vi "CSTK_Button_Icon_Dialog_Configuration.vi"(11 "State in":T1={"ButtonSize"={"False"={"Width"=0, "Height"=0}, "True"={"Width"=0, "Height"=0}, "True to False"={"Width"=0, "Height"=0}, "False to True"={"Width"=0, "Height"=0}, "Hover in False"={"Width"=0, "Height"=0}, "Hover in True"={"Width"=0, "Height"=0}}, "Logo Image"={"False"={"image type"=0, "image depth"=0, "image"=[], "mask"=[], "colors"=[], "Rectangle"={"left"=0, "top"=0, "right"=0, "bottom"=0}}, "True"={"image type"=0, "image depth"=0, "image"=[], "mask"=[], "colors"=[], "Rectangle"={"left"=0, "top"=0, "right"=0, "bottom"=0}}, "True to False"={"image type"=0, "image depth"=0, "image"=[], "mask"=[], "colors"=[], "Rectangle"={"left"=0, "top"=0, "right"=0, "bottom"=0}}, "False to True"={"image type"=0, "image depth"=0, "image"=[], "mask"=[], "colors"=[], "Rectangle"={"left"=0, "top"=0, "right"=0, "bottom"=0}}, "Hover in False"={"image type"=0, "image depth"=0, "image"=[], "mask"=[], "colors"=[], "Rectangle"={"left"=0, "top"=0, "right"=0, "bottom"=0}}, "Hover in True"={"image type"=0, "image depth"=0, "image"=[], "mask"=[], "colors"=[], "Rectangle"={"left"=0, "top"=0, "right"=0, "bottom"=0}}}, "Logo Properties"={"False"={"Display Logo?"=FALSE, "Horizontal Offset"=0}, "True"={"Display Logo?"=FALSE, "Horizontal Offset"=0}, "True to False"={"Display Logo?"=FALSE, "Horizontal Offset"=0}, "False to True"={"Display Logo?"=FALSE, "Horizontal Offset"=0}, "Hover in False"={"Display Logo?"=FALSE, "Horizontal Offset"=0}, "Hover in True"={"Display Logo?"=FALSE, "Horizontal Offset"=0}}, "Text String"={"False"="", "True"="", "True to False"="", "False to True"="", "Hover in False"="", "Hover in True"=""}, "Text Properties"={"False"={"Display Text?"=FALSE, "Text Color"=0, "Horizontal Offset"=0, "Font Style"={"Font Name"="", "Size"=0, "Strikeout?"=FALSE, "Italic?"=FALSE, "Underline?"=FALSE, "Outline?"=FALSE, "Shadow?"=FALSE, "Bold?"=FALSE}}, "True"={"Display Text?"=FALSE, "Text Color"=0, "Horizontal Offset"=0, "Font Style"={"Font Name"="", "Size"=0, "Strikeout?"=FALSE, "Italic?"=FALSE, "Underline?"=FALSE, "Outline?"=FALSE, "Shadow?"=FALSE, "Bold?"=FALSE}}, "True to False"={"Display Text?"=FALSE, "Text Color"=0, "Horizontal Offset"=0, "Font Style"={"Font Name"="", "Size"=0, "Strikeout?"=FALSE, "Italic?"=FALSE, "Underline?"=FALSE, "Outline?"=FALSE, "Shadow?"=FALSE, "Bold?"=FALSE}}, "False to True"={"Display Text?"=FALSE, "Text Color"=0, "Horizontal Offset"=0, "Font Style"={"Font Name"="", "Size"=0, "Strikeout?"=FALSE, "Italic?"=FALSE, "Underline?"=FALSE, "Outline?"=FALSE, "Shadow?"=FALSE, "Bold?"=FALSE}}, "Hover in False"={"Display Text?"=FALSE, "Text Color"=0, "Horizontal Offset"=0, "Font Style"={"Font Name"="", "Size"=0, "Strikeout?"=FALSE, "Italic?"=FALSE, "Underline?"=FALSE, "Outline?"=FALSE, "Shadow?"=FALSE, "Bold?"=FALSE}}, "Hover in True"={"Display Text?"=FALSE, "Text Color"=0, "Horizontal Offset"=0, "Font Style"={"Font Name"="", "Size"=0, "Strikeout?"=FALSE, "Italic?"=FALSE, "Underline?"=FALSE, "Outline?"=FALSE, "Shadow?"=FALSE, "Bold?"=FALSE}}}, "BG Color"={"False"=0, "True"=0, "True to False"=0, "False to True"=0, "Hover in False"=0, "Hover in True"=0}, "Border Color"={"False"=0, "True"=0, "True to False"=0, "False to True"=0, "Hover in False"=0, "Hover in True"=0}, "Border Properties"={"False"={"Radius"=0, "Border Style"={"Width"=3, "Style"=enum."Solid"}}, "True"={"Radius"=0, "Border Style"={"Width"=3, "Style"=enum."Solid"}}, "True to False"={"Radius"=0, "Border Style"={"Width"=3, "Style"=enum."Solid"}}, "False to True"={"Radius"=0, "Border Style"={"Width"=3, "Style"=enum."Solid"}}, "Hover in False"={"Radius"=0, "Border Style"={"Width"=3, "Style"=enum."Solid"}}, "Hover in True"={"Radius"=0, "Border Style"={"Width"=3, "Style"=enum."Solid"}}}, "Current BG Image"={"False"=bytes[0], "True"=bytes[0], "True to False"=bytes[0], "False to True"=bytes[0], "Hover in False"=bytes[0], "Hover in True"=bytes[0]}, "DrawAreaSize"={"False"={"Width"=0, "Height"=0}, "True"={"Width"=0, "Height"=0}, "True to False"={"Width"=0, "Height"=0}, "False to True"={"Width"=0, "Height"=0}, "Hover in False"={"Width"=0, "Height"=0}, "Hover in True"={"Width"=0, "Height"=0}}, "Text String Offset"={"False"=0, "True"=0, "True to False"=0, "False to True"=0, "Hover in False"=0, "Hover in True"=0}} caption="状态") -> (1 "Action Name":string, 2 "State Changed?":bool, 3 "State out":T1={"ButtonSize"={"False"={"Width"=0, "Height"=0}, "True"={"Width"=0, "Height"=0}, "True to False"={"Width"=0, "Height"=0}, "False to True"={"Width"=0, "Height"=0}, "Hover in False"={"Width"=0, "Height"=0}, "Hover in True"={"Width"=0, "Height"=0}}, "Logo Image"={"False"={"image type"=0, "image depth"=0, "image"=[], "mask"=[], "colors"=[], "Rectangle"={"left"=0, "top"=0, "right"=0, "bottom"=0}}, "True"={"image type"=0, "image depth"=0, "image"=[], "mask"=[], "colors"=[], "Rectangle"={"left"=0, "top"=0, "right"=0, "bottom"=0}}, "True to False"={"image type"=0, "image depth"=0, "image"=[], "mask"=[], "colors"=[], "Rectangle"={"left"=0, "top"=0, "right"=0, "bottom"=0}}, "False to True"={"image type"=0, "image depth"=0, "image"=[], "mask"=[], "colors"=[], "Rectangle"={"left"=0, "top"=0, "right"=0, "bottom"=0}}, "Hover in False"={"image type"=0, "image depth"=0, "image"=[], "mask"=[], "colors"=[], "Rectangle"={"left"=0, "top"=0, "right"=0, "bottom"=0}}, "Hover in True"={"image type"=0, "image depth"=0, "image"=[], "mask"=[], "colors"=[], "Rectangle"={"left"=0, "top"=0, "right"=0, "bottom"=0}}}, "Logo Properties"={"False"={"Display Logo?"=FALSE, "Horizontal Offset"=0}, "True"={"Display Logo?"=FALSE, "Horizontal Offset"=0}, "True to False"={"Display Logo?"=FALSE, "Horizontal Offset"=0}, "False to True"={"Display Logo?"=FALSE, "Horizontal Offset"=0}, "Hover in False"={"Display Logo?"=FALSE, "Horizontal Offset"=0}, "Hover in True"={"Display Logo?"=FALSE, "Horizontal Offset"=0}}, "Text String"={"False"="", "True"="", "True to False"="", "False to True"="", "Hover in False"="", "Hover in True"=""}, "Text Properties"={"False"={"Display Text?"=FALSE, "Text Color"=0, "Horizontal Offset"=0, "Font Style"={"Font Name"="", "Size"=0, "Strikeout?"=FALSE, "Italic?"=FALSE, "Underline?"=FALSE, "Outline?"=FALSE, "Shadow?"=FALSE, "Bold?"=FALSE}}, "True"={"Display Text?"=FALSE, "Text Color"=0, "Horizontal Offset"=0, "Font Style"={"Font Name"="", "Size"=0, "Strikeout?"=FALSE, "Italic?"=FALSE, "Underline?"=FALSE, "Outline?"=FALSE, "Shadow?"=FALSE, "Bold?"=FALSE}}, "True to False"={"Display Text?"=FALSE, "Text Color"=0, "Horizontal Offset"=0, "Font Style"={"Font Name"="", "Size"=0, "Strikeout?"=FALSE, "Italic?"=FALSE, "Underline?"=FALSE, "Outline?"=FALSE, "Shadow?"=FALSE, "Bold?"=FALSE}}, "False to True"={"Display Text?"=FALSE, "Text Color"=0, "Horizontal Offset"=0, "Font Style"={"Font Name"="", "Size"=0, "Strikeout?"=FALSE, "Italic?"=FALSE, "Underline?"=FALSE, "Outline?"=FALSE, "Shadow?"=FALSE, "Bold?"=FALSE}}, "Hover in False"={"Display Text?"=FALSE, "Text Color"=0, "Horizontal Offset"=0, "Font Style"={"Font Name"="", "Size"=0, "Strikeout?"=FALSE, "Italic?"=FALSE, "Underline?"=FALSE, "Outline?"=FALSE, "Shadow?"=FALSE, "Bold?"=FALSE}}, "Hover in True"={"Display Text?"=FALSE, "Text Color"=0, "Horizontal Offset"=0, "Font Style"={"Font Name"="", "Size"=0, "Strikeout?"=FALSE, "Italic?"=FALSE, "Underline?"=FALSE, "Outline?"=FALSE, "Shadow?"=FALSE, "Bold?"=FALSE}}}, "BG Color"={"False"=0, "True"=0, "True to False"=0, "False to True"=0, "Hover in False"=0, "Hover in True"=0}, "Border Color"={"False"=0, "True"=0, "True to False"=0, "False to True"=0, "Hover in False"=0, "Hover in True"=0}, "Border Properties"={"False"={"Radius"=0, "Border Style"={"Width"=3, "Style"=enum."Solid"}}, "True"={"Radius"=0, "Border Style"={"Width"=3, "Style"=enum."Solid"}}, "True to False"={"Radius"=0, "Border Style"={"Width"=3, "Style"=enum."Solid"}}, "False to True"={"Radius"=0, "Border Style"={"Width"=3, "Style"=enum."Solid"}}, "Hover in False"={"Radius"=0, "Border Style"={"Width"=3, "Style"=enum."Solid"}}, "Hover in True"={"Radius"=0, "Border Style"={"Width"=3, "Style"=enum."Solid"}}}, "Current BG Image"={"False"=bytes[0], "True"=bytes[0], "True to False"=bytes[0], "False to True"=bytes[0], "Hover in False"=bytes[0], "Hover in True"=bytes[0]}, "DrawAreaSize"={"False"={"Width"=0, "Height"=0}, "True"={"Width"=0, "Height"=0}, "True to False"={"Width"=0, "Height"=0}, "False to True"={"Width"=0, "Height"=0}, "Hover in False"={"Width"=0, "Height"=0}, "Hover in True"={"Width"=0, "Height"=0}}, "Text String Offset"={"False"=0, "True"=0, "True to False"=0, "False to True"=0, "Hover in False"=0, "Hover in True"=0}} caption="状态")   [LabVIEW 2015, in "CSTK_Button_Icon.xctl"]
uses:
  CSTK_Button_Icon.xctl
  Private/TypeDefinitions/CSTK_Button_Icon_Properties_Configure.ctl
  Private/TypeDefinitions/_CSTK_Button_Icon_TextProperties_FontStyle.ctl
  CSTK_Button_Icon_Status.ctl
  Private/TypeDefinitions/_CSTK_Button_Icon_ButtonSize.ctl
  <vilib>/Utility/miscctls.llb/LVBoundsTypeDef.ctl
  Private/TypeDefinitions/_CSTK_Button_Icon_LogoImage.ctl
  <vilib>/picture/picture.llb/imagedata.ctl
  Private/TypeDefinitions/_CSTK_Button_Icon_LogoProperties.ctl
  Private/TypeDefinitions/_CSTK_Button_Icon_LogoProperties_Data.ctl
  Private/TypeDefinitions/_CSTK_Button_Icon_TextString.ctl
  Private/TypeDefinitions/_CSTK_Button_Icon_TextProperties.ctl
  Private/TypeDefinitions/_CSTK_Button_Icon_TextProperties_Data.ctl
  Private/TypeDefinitions/_CSTK_Button_Icon_BGColor.ctl
  Private/TypeDefinitions/_CSTK_Button_Icon_BorderColor.ctl
  Private/TypeDefinitions/_CSTK_Button_Icon_BorderProperties.ctl
  Private/TypeDefinitions/_CSTK_Button_Icon_BorderProperties_Data.ctl
  Private/TypeDefinitions/_CSTK_Button_Icon_CurrentBGImage.ctl
  Private/TypeDefinitions/_CSTK_Button_Icon_DrawAreaSize.ctl
  Private/TypeDefinitions/_CSTK_Button_Icon_TextStartOffset.ctl
  <vilib>/Utility/miscctls.llb/LVPointTypeDef.ctl
panel:
  in  "放大比例":dbl(slide) scale=0.0..2.0 scale format="%#.2f"
  in  "选项卡控件":T19(tab)
  in  "cfg_False":T20={"背景颜色"=0, "LOGO"={"显示LOGO"=FALSE, "水平偏移"=0, "LOGO路径"=path "", "LOGO图片"=bytes[0]}, "布尔文本"={"显示文本"=FALSE, "水平偏移"=0, "布尔文本"="", "文本颜色"=0, "字体样式"={"Font Name"="", "Size"=17, "Strikeout?"=FALSE, "Italic?"=FALSE, "Underline?"=FALSE, "Outline?"=FALSE, "Shadow?"=FALSE, "Bold?"=FALSE}}, "边框"={"颜色"=0, "线条宽度"=0, "圆角半径"=0, "线条样式"=enum."Solid"}}
  in  "cfg_True":T20={"背景颜色"=0, "LOGO"={"显示LOGO"=FALSE, "水平偏移"=0, "LOGO路径"=path "", "LOGO图片"=bytes[0]}, "布尔文本"={"显示文本"=FALSE, "水平偏移"=0, "布尔文本"="", "文本颜色"=0, "字体样式"={"Font Name"="", "Size"=17, "Strikeout?"=FALSE, "Italic?"=FALSE, "Underline?"=FALSE, "Outline?"=FALSE, "Shadow?"=FALSE, "Bold?"=FALSE}}, "边框"={"颜色"=0, "线条宽度"=0, "圆角半径"=0, "线条样式"=enum."Solid"}}
  in  "cfg_TrueToFalse":T20={"背景颜色"=0, "LOGO"={"显示LOGO"=FALSE, "水平偏移"=0, "LOGO路径"=path "", "LOGO图片"=bytes[0]}, "布尔文本"={"显示文本"=FALSE, "水平偏移"=0, "布尔文本"="", "文本颜色"=0, "字体样式"={"Font Name"="", "Size"=17, "Strikeout?"=FALSE, "Italic?"=FALSE, "Underline?"=FALSE, "Outline?"=FALSE, "Shadow?"=FALSE, "Bold?"=FALSE}}, "边框"={"颜色"=0, "线条宽度"=0, "圆角半径"=0, "线条样式"=enum."Solid"}}
  in  "cfg_FalseToTrue":T20={"背景颜色"=0, "LOGO"={"显示LOGO"=FALSE, "水平偏移"=0, "LOGO路径"=path "", "LOGO图片"=bytes[0]}, "布尔文本"={"显示文本"=FALSE, "水平偏移"=0, "布尔文本"="", "文本颜色"=0, "字体样式"={"Font Name"="", "Size"=17, "Strikeout?"=FALSE, "Italic?"=FALSE, "Underline?"=FALSE, "Outline?"=FALSE, "Shadow?"=FALSE, "Bold?"=FALSE}}, "边框"={"颜色"=0, "线条宽度"=0, "圆角半径"=0, "线条样式"=enum."Solid"}}
  in  "cfg_HoverInFalse":T20={"背景颜色"=0, "LOGO"={"显示LOGO"=FALSE, "水平偏移"=0, "LOGO路径"=path "", "LOGO图片"=bytes[0]}, "布尔文本"={"显示文本"=FALSE, "水平偏移"=0, "布尔文本"="", "文本颜色"=0, "字体样式"={"Font Name"="", "Size"=17, "Strikeout?"=FALSE, "Italic?"=FALSE, "Underline?"=FALSE, "Outline?"=FALSE, "Shadow?"=FALSE, "Bold?"=FALSE}}, "边框"={"颜色"=0, "线条宽度"=0, "圆角半径"=0, "线条样式"=enum."Solid"}}
  in  "cfg_HoverInTrue":T20={"背景颜色"=0, "LOGO"={"显示LOGO"=FALSE, "水平偏移"=0, "LOGO路径"=path "", "LOGO图片"=bytes[0]}, "布尔文本"={"显示文本"=FALSE, "水平偏移"=0, "布尔文本"="", "文本颜色"=0, "字体样式"={"Font Name"="", "Size"=17, "Strikeout?"=FALSE, "Italic?"=FALSE, "Underline?"=FALSE, "Outline?"=FALSE, "Shadow?"=FALSE, "Bold?"=FALSE}}, "边框"={"颜色"=0, "线条宽度"=0, "圆角半径"=0, "线条样式"=enum."Solid"}}
  out "预览":picture
  in  "修改模式":enum16{"单独修改各状态", "统一修改T/F状态", "统一修改全部状态"}(ring)
  in  "按钮大小":cluster{"Width":u32, "Height":u32}
  in  "取消按钮":bool
  in  "确定按钮":bool
  # "Button Icon Configuration"
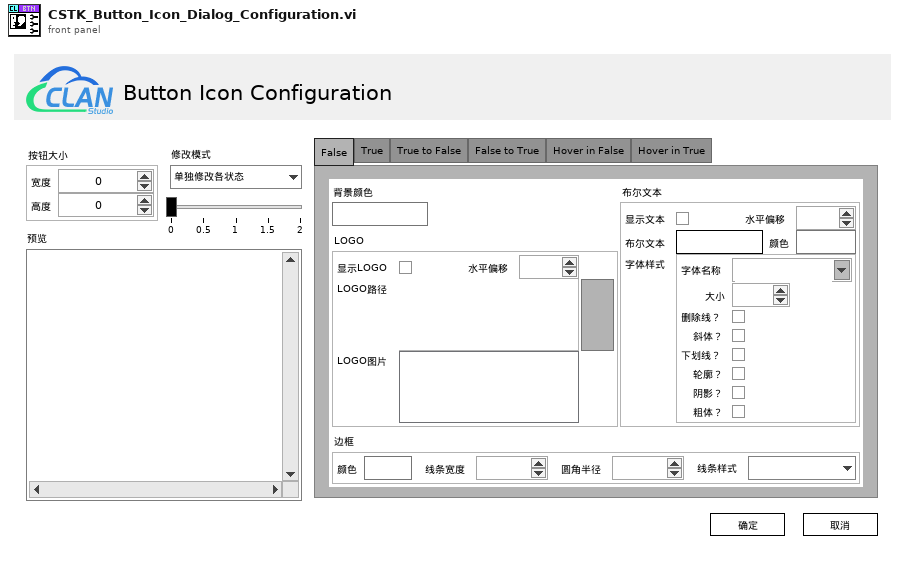
[diagram p1: front panel]
types:
  T1 = typedef "CSTK_Button_Icon.xctl/CSTK_Button_Icon_Status.ctl" = cluster{"ButtonSize":T2, "Logo Image":T4, "Logo Properties":T6, "Text String":T8, "Text Properties":T9, "BG Color":T12, "Border Color":T13, "Border Properties":T14, "Current BG Image":T16, "DrawAreaSize":T17, "Text String Offset":T18}
  T2 = typedef "CSTK_Button_Icon.xctl/_CSTK_Button_Icon_ButtonSize.ctl" = cluster{"False":T3, "True":T3, "True to False":T3, "False to True":T3, "Hover in False":T3, "Hover in True":T3}
  T3 = typedef "LVBoundsTypeDef.ctl" = cluster{"Width":u32, "Height":u32}
  T4 = typedef "CSTK_Button_Icon.xctl/_CSTK_Button_Icon_LogoImage.ctl" = cluster{"False":T5, "True":T5, "True to False":T5, "False to True":T5, "Hover in False":T5, "Hover in True":T5}
  T5 = typedef "imagedata.ctl" = cluster{"image type":i32, "image depth":i32, "image":u8[], "mask":u8[], "colors":u32[], "Rectangle":cluster{"left":i16, "top":i16, "right":i16, "bottom":i16}}
  T6 = typedef "CSTK_Button_Icon.xctl/_CSTK_Button_Icon_LogoProperties.ctl" = cluster{"False":T7, "True":T7, "True to False":T7, "False to True":T7, "Hover in False":T7, "Hover in True":T7}
  T7 = typedef "CSTK_Button_Icon.xctl/_CSTK_Button_Icon_LogoProperties_Data.ctl" = cluster{"Display Logo?":bool, "Horizontal Offset":i16}
  T8 = typedef "CSTK_Button_Icon.xctl/_CSTK_Button_Icon_TextString.ctl" = cluster{"False":string, "True":string, "True to False":string, "False to True":string, "Hover in False":string, "Hover in True":string}
  T9 = typedef "CSTK_Button_Icon.xctl/_CSTK_Button_Icon_TextProperties.ctl" = cluster{"False":T10, "True":T10, "True to False":T10, "False to True":T10, "Hover in False":T10, "Hover in True":T10}
  T10 = typedef "CSTK_Button_Icon.xctl/_CSTK_Button_Icon_TextProperties_Data.ctl" = cluster{"Display Text?":bool, "Text Color":u32, "Horizontal Offset":i16, "Font Style":T11}
  T11 = typedef "CSTK_Button_Icon.xctl/_CSTK_Button_Icon_TextProperties_FontStyle.ctl" = cluster{"Font Name":string, "Size":i16, "Strikeout?":bool, "Italic?":bool, "Underline?":bool, "Outline?":bool, "Shadow?":bool, "Bold?":bool}
  T12 = typedef "CSTK_Button_Icon.xctl/_CSTK_Button_Icon_BGColor.ctl" = cluster{"False":u32, "True":u32, "True to False":u32, "False to True":u32, "Hover in False":u32, "Hover in True":u32}
  T13 = typedef "CSTK_Button_Icon.xctl/_CSTK_Button_Icon_BorderColor.ctl" = cluster{"False":u32, "True":u32, "True to False":u32, "False to True":u32, "Hover in False":u32, "Hover in True":u32}
  T14 = typedef "CSTK_Button_Icon.xctl/_CSTK_Button_Icon_BorderProperties.ctl" = cluster{"False":T15, "True":T15, "True to False":T15, "False to True":T15, "Hover in False":T15, "Hover in True":T15}
  T15 = typedef "CSTK_Button_Icon.xctl/_CSTK_Button_Icon_BorderProperties_Data.ctl" = cluster{"Radius":i16, "Border Style":cluster{"Width":u16, "Style":enum32{"Solid", "Dash", "Dot", "DashDot", "DashDotDot"}}}
  T16 = typedef "CSTK_Button_Icon.xctl/_CSTK_Button_Icon_CurrentBGImage.ctl" = cluster{"False":picture, "True":picture, "True to False":picture, "False to True":picture, "Hover in False":picture, "Hover in True":picture}
  T17 = typedef "CSTK_Button_Icon.xctl/_CSTK_Button_Icon_DrawAreaSize.ctl" = cluster{"False":T3, "True":T3, "True to False":T3, "False to True":T3, "Hover in False":T3, "Hover in True":T3}
  T18 = typedef "CSTK_Button_Icon.xctl/_CSTK_Button_Icon_TextStartOffset.ctl" = cluster{"False":i32, "True":i32, "True to False":i32, "False to True":i32, "Hover in False":i32, "Hover in True":i32}
  T19 = enum32{"False", "True", "True to False", "False to True", "Hover in False", "Hover in True"}
  T20 = typedef "CSTK_Button_Icon.xctl/CSTK_Button_Icon_Properties_Configure.ctl" = cluster{"背景颜色":u32, "LOGO":cluster{"显示LOGO":bool, "水平偏移":i16, "LOGO路径":path, "LOGO图片":picture}, "布尔文本":cluster{"显示文本":bool, "水平偏移":i16, "布尔文本":string, "文本颜色":u32, "字体样式":T11}, "边框":cluster{"颜色":u32, "线条宽度":u16, "圆角半径":i16, "线条样式":enum32{"Solid", "Dash", "Dot", "DashDot", "DashDotDot"}}}
  T21 = cluster{"Action":string, "Value":variant, "Remark":string}[]
  T22 = enum32{"Invalid", "Standard", "Closed", "Hidden", "Minimized", "Maximized"}
  T23 = cluster{"Action":string, "Value":variant, "Remark":string}
  T24 = typedef "LVPointTypeDef.ctl" = cluster{"Horizontal":i16, "Vertical":i16}
  T25 = typedef "eventvkey.ctl" = enum16{"ASCII", "Enter", "Return", "Shift", "Ctrl", "Alt", "Cmd", "Opt", "Caps", "NumLock", "Clear", "Break", "Up", "Down", "Left", "Right", "Insert", "Delete", "Home", "End", "PageUp", "PageDown", "Escape", "Help", "Pause", "ScrollLock", "F1", "F2", "F3", "F4", "F5", "F6", "F7", "F8", "F9", "F10", "F11", "F12", "F13", "F14", "F15", "F16", "F17", "F18", "F19", "F20", "F21", "F22", "F23", "F24", "Play", "VolumeUp", "VolumeDown", "Mute", "Two Byte Char"}
  T26 = cluster{"Shift":bool, "Ctrl":bool, "Alt":bool, "Cmd":bool, "Opt":bool}
  T27 = cluster{"[0]":cluster{"Width":u32, "Height":u32}, "[1]":cluster{"Width":u32, "Height":u32}, "[2]":cluster{"Width":u32, "Height":u32}, "[3]":cluster{"Width":u32, "Height":u32}, "[4]":cluster{"Width":u32, "Height":u32}, "[5]":cluster{"Width":u32, "Height":u32}}
  T28 = enum32{"Page Enabled", "Page Disabled", "Page Disabled & Grayed"}[]
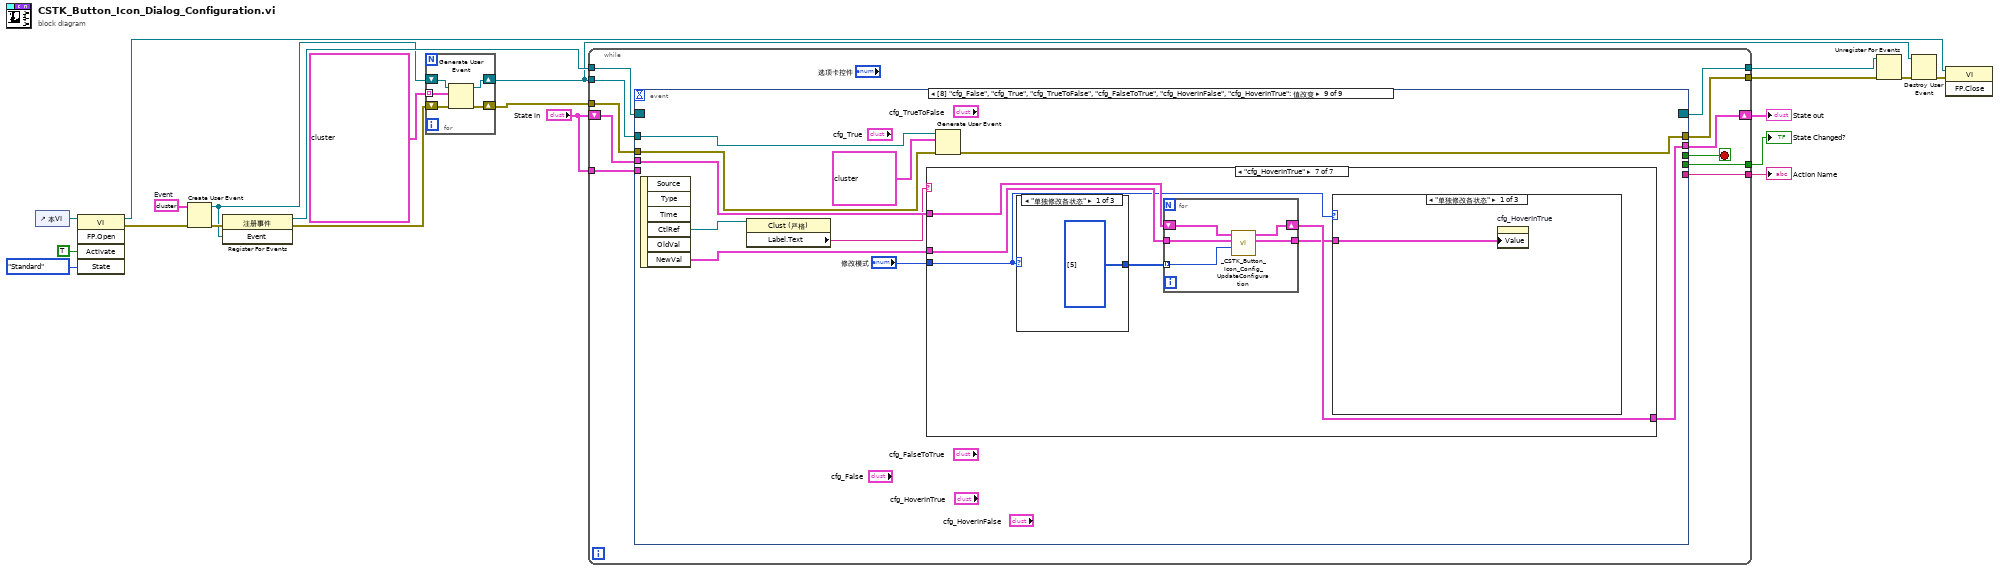
[diagram p0: block diagram]
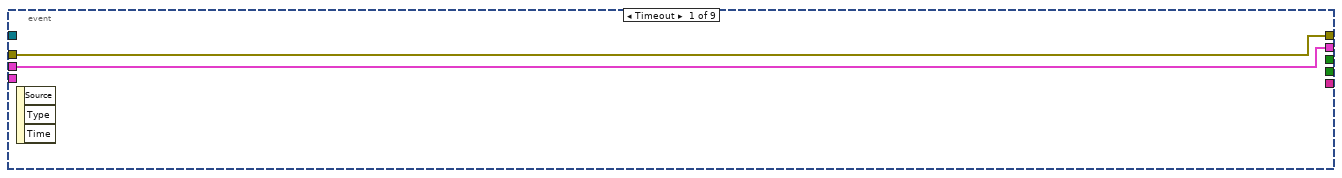
[diagram p2: hidden frame]
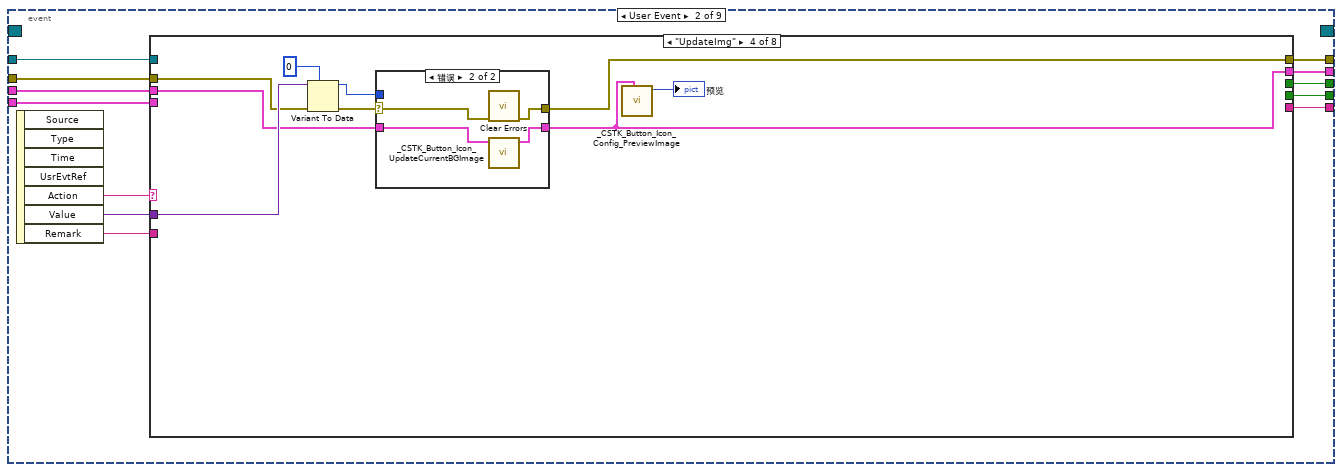
[diagram p3: hidden frame]
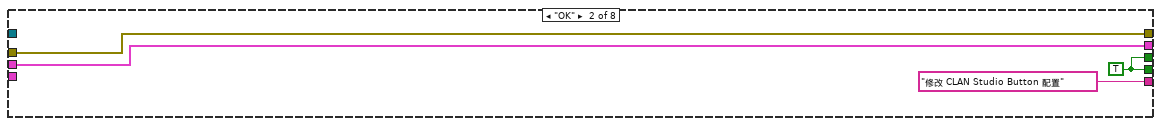
[diagram p5: hidden frame]
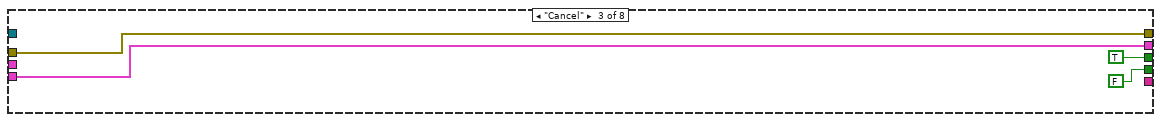
[diagram p6: hidden frame]
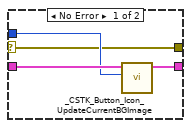
[diagram p7: hidden frame]
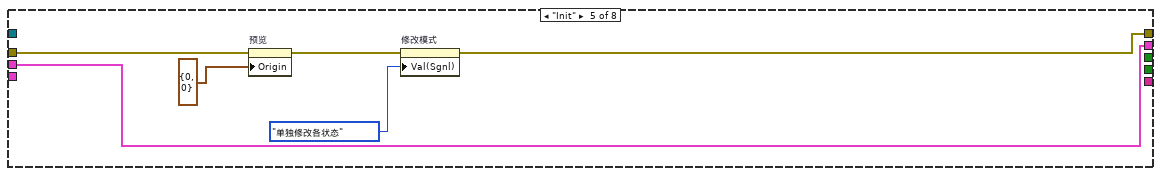
[diagram p8: hidden frame]
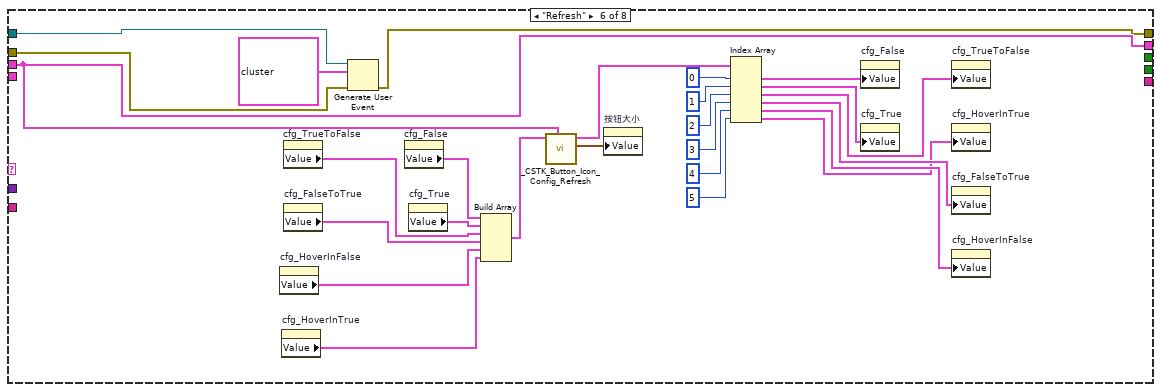
[diagram p9: hidden frame]
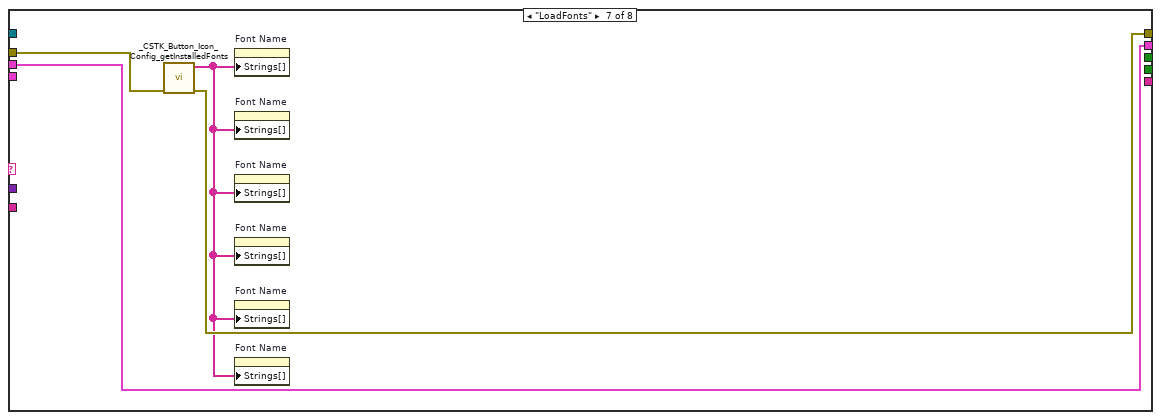
[diagram p10: hidden frame]
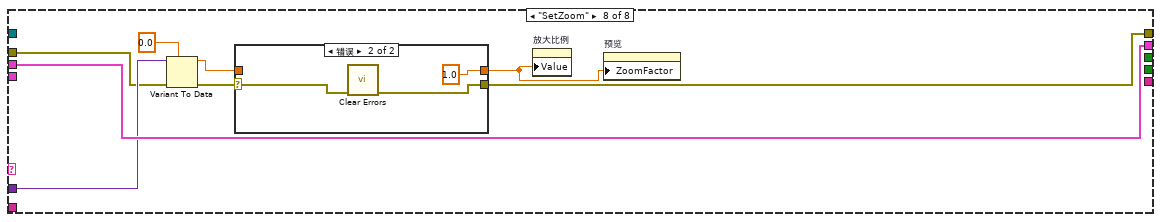
[diagram p11: hidden frame]
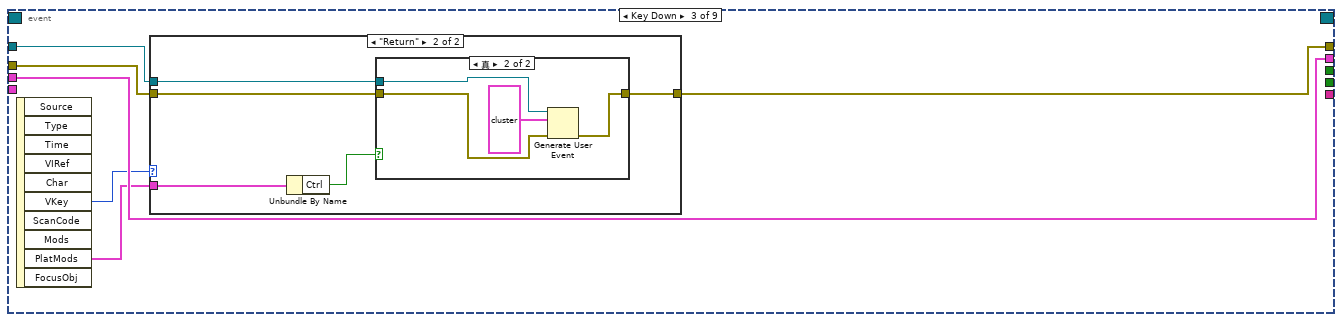
[diagram p13: hidden frame]
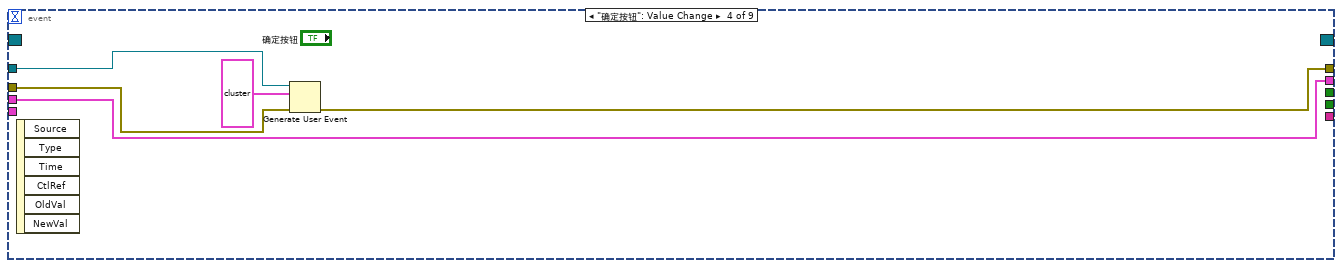
[diagram p16: hidden frame]
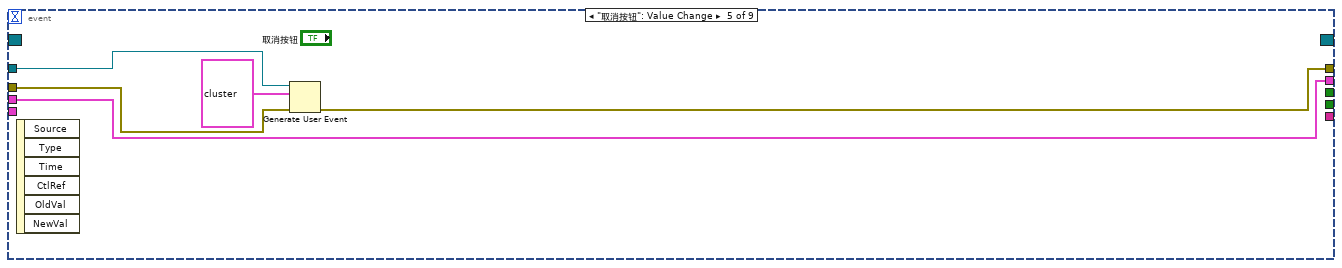
[diagram p17: hidden frame]
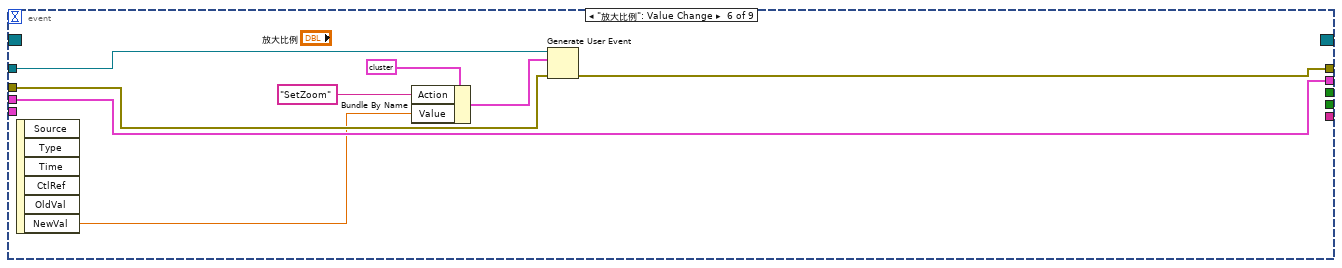
[diagram p18: hidden frame]
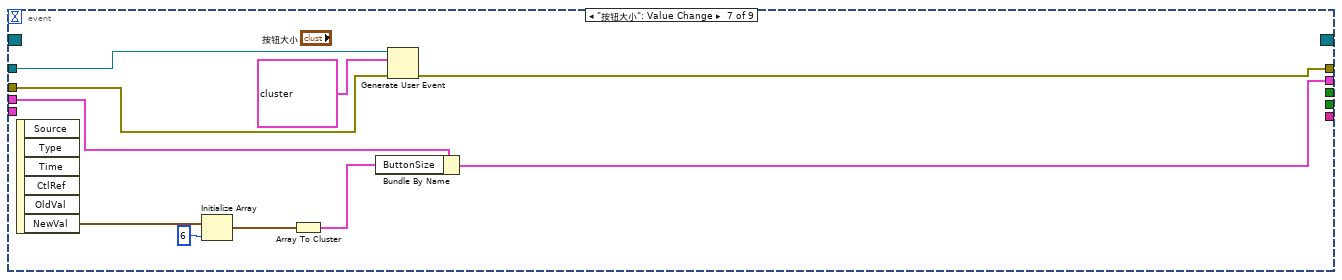
[diagram p19: hidden frame]
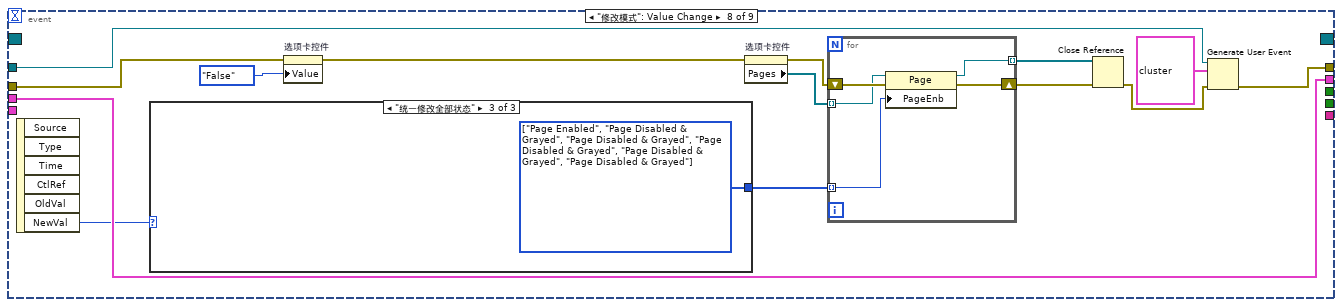
[diagram p20: hidden frame]
diagram:
  w19 = T23 {"Action"="", "Value"=variant, "Remark"=""}  # Event
  n1 = control-ref of="本VI"() -> (w10:refnum<vi>)
  n2 = invoke class="VI" method="FP.Open"(reference=w10, "Activate"=TRUE ("激活？"), "State"=T22."Standard" ("状态")) -> (reference out=w5:refnum<vi>, error out=w7:errorcluster)  [unwired: 2 in, 3 out]
  n3 = Create User Event(user event datatype=w19, error in=w7) -> (user event=w3:refnum<user-event>, error out=w20:errorcluster)
  n4 = register-events(error in=w20, w3) -> (reference out=w21:refnum<event-registration>, error out=w4:errorcluster)  [unwired: 1 in]
  n5 = for {
    shift-right: [w26] -> w18
    shift-left: w4 -> [w24]
    shift-right: [w25] -> w14
    shift-left: w3 -> [w23]
    tunnel: T21 [{"Action"="Init", "Value"=variant, "Remark"=""}, {"Action"="SetZoom", "Value"=variant, "Remark"=""}, {"Action"="LoadFonts", "Value"=variant, "Remark"=""}, {"Action"="Refresh", "Value"=variant, "Remark"=""}] ("事件数据") -> [w22] mode=indexing
    n6 = Generate User Event(user event=w23, event data cluster=w22, error in=w24) -> (user event out=w25:refnum<user-event>, error out=w26:errorcluster)  [unwired: 1 in]
  }
  n7 = while {
    shift-right: [w36] -> w1
    shift-left: "State in" -> [w37]
    tunnel: w21 -> [w35]
    tunnel: w14 -> [w34]
    tunnel: w18 -> [w31]
    tunnel: [w33] -> w16
    tunnel: [w32] -> w15
    tunnel: [w29] -> w13
    tunnel: "State in" -> [w28]
    tunnel: [w27] -> w11
    stop <- w30 stop-if-true
    n8 = event shown="[8] \"cfg_False\", \"cfg_True\", \"cfg_TrueToFalse\", \"cfg_FalseToTrue\", \"cfg_HoverInFalse\", \"cfg_HoverInTrue\": 值改变" {
      selector: w35 -> [_ _ _ _ _ _ _ _ _]
      dyn-events: [_ _ _ _ _ _ _ _ _] -> w33
      timeout: _ -> [_ _ _ _ _ _ _ _ _]
      tunnel: w37 -> [w39 w48 w133 w149 w154 w162 w172 w186 w202]
      tunnel: [w39 w47 w133 w149 w154 w162 w171 w186 w203] -> w36
      tunnel: w34 -> [_ w40 w128 w146 w151 w159 w164 w174 w198]
      tunnel: [w38 w49 w129 w147 w152 w160 w163 w175 w195] -> w32
      tunnel: w31 -> [w38 w50 w130 w148 w153 w161 w165 w178 w196]
      tunnel: [_ w46 _ _ _ _ _ _ _] -> w30
      tunnel: [_ w45 _ _ _ _ _ _ _] -> w29
      tunnel: w28 -> [_ w44 _ _ _ _ _ _ _]
      tunnel: [_ w43 _ _ _ _ _ _ _] -> w27
      event Timeout {
        n9 = event-data() -> ()  [unwired: 1 in, 3 out]
      }
      event User Event {
        n10 = event-data() -> ("Action"=w51:string, "Value"=w42:variant, "Remark"=w41:string)  [unwired: 1 in, 4 out]
        n11 = case shown="\"UpdateImg\"" w51 {
          tunnel: [w53 w57 w61 w64 w80 w94 w112 w116] -> w49
          tunnel: w50 -> [w53 w57 w61 w68 w81 w95 w113 w117]
          tunnel: [w52 w56 w58 w62 w84 w110 w114 w122] -> w47
          tunnel: w48 -> [w52 w56 _ w65 w84 w110 w114 w122]
          tunnel: [_ w55 TRUE _ _ _ _ _] -> w46
          tunnel: [_ w55 FALSE _ _ _ _ _] -> w45
          tunnel: w44 -> [_ _ w58 _ _ _ _ _]
          tunnel: [_ "修改 CLAN Studio Button 配置" _ _ _ _ _ _] -> w43
          tunnel: w42 -> [_ _ _ w69 _ _ _ w118]
          tunnel: w41 -> [_ _ _ _ _ _ _ _]
          tunnel: w40 -> [_ _ _ _ _ w93 _ _]
          frame Default {
          }
          frame "OK" {
            w55 = TRUE
          }
          frame "Cancel" {
          }
          frame "UpdateImg" {
            n12 = Variant To Data(error in=w68, type=0, Variant=w69) -> (data=w66:i32, error out=w67:errorcluster)
            n13 = case shown="错误" w67 {
              selector: w67 -> [w71 w78]
              tunnel: w66 -> [w72 _]
              tunnel: w65 -> [w74 w77]
              tunnel: [w73 w76] -> w62
              tunnel: [w71 w75] -> w64
              frame No Error {
                n14 = call "_CSTK_Button_Icon_UpdateCurrentBGImage.vi"("Update Index (ALL:-1)"=w72, "State in"=w74) -> ("State out"=w73:T1)  [unwired: 9 in]
              }
              frame Error {
                n15 = call <vilib>:"Clear Errors.vi"("error in (no error)"=w78) -> ("error out"=w75:errorcluster)  [unwired: 5 in, 1 out]
                n16 = call "_CSTK_Button_Icon_UpdateCurrentBGImage.vi"("State in"=w77) -> ("State out"=w76:T1)  [unwired: 10 in]
              }
            }
            n17 = call "_CSTK_Button_Icon_Config_PreviewImage.vi"("State in"=w62) -> ("Preview Image"=→"预览":picture)  [unwired: 10 in]
          }
          frame "Init" {
            n18 = property on="预览" class="Pict"(error in=w81, "Origin"=T24 {"Horizontal"=0, "Vertical"=0} ("原点")) -> (error out=w82:errorcluster)  [unwired: 1 in, 1 out]
            n19 = property on="修改模式" class="Enum (严格)"(error in=w82, "Val(Sgnl)"=enum16{"单独修改各状态", "统一修改T/F状态", "统一修改全部状态"}."单独修改各状态" ("值(信号)")) -> (error out=w80:errorcluster)  [unwired: 1 in, 1 out]
          }
          frame "Refresh" {
            n20 = property on="cfg_HoverInFalse" class="Clust (严格)"() -> ("Value"=w87:T20)  [unwired: 2 in, 2 out]
            n21 = property on="cfg_HoverInTrue" class="Clust (严格)"() -> ("Value"=w86:T20)  [unwired: 2 in, 2 out]
            n22 = property on="cfg_TrueToFalse" class="Clust (严格)"() -> ("Value"=w89:T20)  [unwired: 2 in, 2 out]
            n23 = property on="cfg_FalseToTrue" class="Clust (严格)"() -> ("Value"=w88:T20)  [unwired: 2 in, 2 out]
            n24 = Generate User Event(user event=w93, event data cluster=T23 {"Action"="UpdateImg", "Value"=variant, "Remark"=""} ("事件数据"), error in=w95) -> (error out=w94:errorcluster)  [unwired: 1 in, 1 out]
            n25 = property on="cfg_False" class="Clust (严格)"() -> ("Value"=w91:T20)  [unwired: 2 in, 2 out]
            n26 = property on="cfg_True" class="Clust (严格)"() -> ("Value"=w90:T20)  [unwired: 2 in, 2 out]
            n27 = Build Array(w91, w90, w89, w88, w87, w86) -> (w85:T20[])
            n28 = call "_CSTK_Button_Icon_Config_Refresh.vi"("State in"=w110, "Configuration in"=w85) -> ("按钮大小"=w109:cluster{"Width":u32, "Height":u32}, "Configuration out"=w108:T20[])  [unwired: 8 in]
            n29 = property on="按钮大小" class="Clust (严格)"("Value"=w109) -> ()  [unwired: 2 in, 2 out]
            n30 = Index Array(array=w108, index #1=0 ("索引"), index #2=1 ("索引"), index #3=2 ("索引"), index #4=3 ("索引"), index #5=4 ("索引"), index #6=5 ("索引")) -> (element #1=w101:T20, element #2=w100:T20, element #3=w99:T20, element #4=w98:T20, element #5=w97:T20, element #6=w96:T20)
            n31 = property on="cfg_False" class="Clust (严格)"("Value"=w101) -> ()  [unwired: 2 in, 2 out]
            n32 = property on="cfg_True" class="Clust (严格)"("Value"=w100) -> ()  [unwired: 2 in, 2 out]
            n33 = property on="cfg_TrueToFalse" class="Clust (严格)"("Value"=w99) -> ()  [unwired: 2 in, 2 out]
            n34 = property on="cfg_HoverInTrue" class="Clust (严格)"("Value"=w96) -> ()  [unwired: 2 in, 2 out]
            n35 = property on="cfg_FalseToTrue" class="Clust (严格)"("Value"=w98) -> ()  [unwired: 2 in, 2 out]
            n36 = property on="cfg_HoverInFalse" class="Clust (严格)"("Value"=w97) -> ()  [unwired: 2 in, 2 out]
          }
          frame "LoadFonts" {
            n37 = call "_CSTK_Button_Icon_Config_getInstalledFonts.vi"("错误输入（无错误）"=w113) -> ("错误输出"=w112:errorcluster, "已安装字体列表"=w111:string[])  [unwired: 9 in]
            n38 = property on="Font Name" class="CmbBox"("Strings[]"=w111) -> ()  [unwired: 2 in, 2 out]
            n39 = property on="Font Name" class="CmbBox"("Strings[]"=w111) -> ()  [unwired: 2 in, 2 out]
            n40 = property on="Font Name" class="CmbBox"("Strings[]"=w111) -> ()  [unwired: 2 in, 2 out]
            n41 = property on="Font Name" class="CmbBox"("Strings[]"=w111) -> ()  [unwired: 2 in, 2 out]
            n42 = property on="Font Name" class="CmbBox"("Strings[]"=w111) -> ()  [unwired: 2 in, 2 out]
            n43 = property on="Font Name" class="CmbBox"("Strings[]"=w111) -> ()  [unwired: 2 in, 2 out]
          }
          frame "SetZoom" {
            n44 = Variant To Data(error in=w117, type=0.0, Variant=w118) -> (data=w119:dbl, error out=w120:errorcluster)
            n45 = case shown="错误" w120 {
              selector: w120 -> [w124 w127]
              tunnel: w119 -> [w123 _]
              tunnel: [w124 w126] -> w116
              tunnel: [w123 1.0] -> w115
              frame No Error {
              }
              frame Error {
                n46 = call <vilib>:"Clear Errors.vi"("error in (no error)"=w127) -> ("error out"=w126:errorcluster)  [unwired: 5 in, 1 out]
              }
            }
            n47 = property on="放大比例" class="Slide (严格)"("Value"=w115) -> ()  [unwired: 2 in, 2 out]
            n48 = property on="预览" class="Pict"("ZoomFactor"=w115) -> ()  [unwired: 2 in, 2 out]
          }
        }
      }
      event Key Down {
        n49 = event-data() -> ("VKey"=w132:T25, "PlatMods"=w131:T26)  [unwired: 1 in, 8 out]
        n50 = case shown="\"Return\"" w132 {
          tunnel: w131 -> [_ w139]
          tunnel: [w134 w137] -> w129
          tunnel: w130 -> [w134 w136]
          tunnel: w128 -> [_ w135]
          frame Default {
          }
          frame "Return" {
            n51 = Unbundle By Name(w139) -> ("Ctrl"=w138:bool)
            n52 = case shown="真" w138 {
              tunnel: [w140 w142] -> w137
              tunnel: w136 -> [w140 w143]
              tunnel: w135 -> [_ w141]
              frame False {
              }
              frame True {
                n53 = Generate User Event(user event=w141, event data cluster=T23 {"Action"="OK", "Value"=variant, "Remark"=""} ("事件数据"), error in=w143) -> (error out=w142:errorcluster)  [unwired: 1 in, 1 out]
              }
            }
          }
        }
      }
      event "确定按钮": Value Change {
        n54 = event-data() -> ()  [unwired: 1 in, 6 out]
        n55 = Generate User Event(user event=w146, event data cluster=T23 {"Action"="OK", "Value"=variant, "Remark"=""} ("事件数据"), error in=w148) -> (error out=w147:errorcluster)  [unwired: 1 in, 1 out]
      }
      event "取消按钮": Value Change {
        n56 = event-data() -> ()  [unwired: 1 in, 6 out]
        n57 = Generate User Event(user event=w151, event data cluster=T23 {"Action"="Cancel", "Value"=variant, "Remark"=""} ("事件数据"), error in=w153) -> (error out=w152:errorcluster)  [unwired: 1 in, 1 out]
      }
      event "放大比例": Value Change {
        n58 = event-data() -> ("NewVal"=w155:dbl)  [unwired: 1 in, 5 out]
        n59 = Bundle By Name(cluster=T23 {"Action"="", "Value"=variant, "Remark"=""} ("事件数据"), "Action"="SetZoom", "Value"=w155) -> (w157:T23)
        n60 = Generate User Event(user event=w159, event data cluster=w157, error in=w161) -> (error out=w160:errorcluster)  [unwired: 1 in, 1 out]
      }
      event "按钮大小": Value Change {
        n61 = event-data() -> ("NewVal"=w167:cluster{"Width":u32, "Height":u32})  [unwired: 1 in, 5 out]
        n62 = Initialize Array(w167, 6 ("维数大小")) -> (w169:cluster{"Width":u32, "Height":u32}[])
        n63 = Array To Cluster(array=w169) -> (cluster=w168:T27)
        n64 = Bundle By Name(cluster=w172, "ButtonSize"=w168) -> (w171:T1)
        n65 = Generate User Event(user event=w164, event data cluster=T23 {"Action"="UpdateImg", "Value"=variant, "Remark"=""} ("事件数据"), error in=w165) -> (error out=w163:errorcluster)  [unwired: 1 in, 1 out]
      }
      event "修改模式": Value Change {
        n66 = event-data() -> ("NewVal"=w177:enum16{"单独修改各状态", "统一修改T/F状态", "统一修改全部状态"})  [unwired: 1 in, 5 out]
        n67 = case shown="\"统一修改全部状态\"" w177 {
          tunnel: [w187 w188 w189] -> w181
          frame "单独修改各状态" {
            w187 = T28 [enum."Page Enabled", enum."Page Enabled", enum."Page Enabled", enum."Page Enabled", enum."Page Enabled", enum."Page Enabled"] items=["Page Enabled", "Page Disabled", "Page Disabled & Grayed"] ("选项卡页启用状态")
          }
          frame "统一修改T/F状态" {
            w188 = T28 [enum."Page Enabled", enum."Page Enabled", enum."Page Disabled & Grayed", enum."Page Disabled & Grayed", enum."Page Disabled & Grayed", enum."Page Disabled & Grayed"] items=["Page Enabled", "Page Disabled", "Page Disabled & Grayed"] ("选项卡页启用状态")
          }
          frame "统一修改全部状态" {
            w189 = T28 [enum."Page Enabled", enum."Page Disabled & Grayed", enum."Page Disabled & Grayed", enum."Page Disabled & Grayed", enum."Page Disabled & Grayed", enum."Page Disabled & Grayed"] items=["Page Enabled", "Page Disabled", "Page Disabled & Grayed"] ("选项卡页启用状态")
          }
        }
        n68 = property on="选项卡控件" class="TabCtl (严格)"(error in=w178, "Value"=T19."False" ("选项卡控件")) -> (error out=w184:errorcluster)  [unwired: 1 in, 1 out]
        n69 = property on="选项卡控件" class="TabCtl (严格)"(error in=w184) -> (error out=w183:errorcluster, "Pages"=w182:refnum<vi>[])  [unwired: 1 in, 1 out]
        n70 = for {
          shift-right: [w192] -> w180
          shift-left: w183 -> [w194]
          tunnel: w182 -> [w193] mode=indexing
          tunnel: w181 -> [w190] mode=indexing
          tunnel: [w191] -> w179 mode=indexing
          n71 = property class="Page"(reference=w193, error in=w194, "PageEnb"=w190) -> (reference out=w191:refnum<vi>, error out=w192:errorcluster)
        }
        n72 = Close Reference(reference=w179, error in (no error)=w180) -> (error out=w176:errorcluster)
        n73 = Generate User Event(user event=w174, event data cluster=T23 {"Action"="Refresh", "Value"=variant, "Remark"=""} ("事件数据"), error in=w176) -> (error out=w175:errorcluster)  [unwired: 1 in, 1 out]
      }
      event Value Change {
        n74 = event-data() -> ("CtlRef"=w204:refnum<vi>, "NewVal"=w201:T20)  [unwired: 1 in, 4 out]
        n75 = property class="Clust (严格)"(reference=w204) -> ("Label.Text"=w200:string)  [unwired: 1 in, 2 out]
        n76 = case shown="\"cfg_HoverInTrue\"" w200 {
          tunnel: [w205 w211 w228 w245 w262 w279 w296] -> w203
          tunnel: w202 -> [w205 w210 w227 w244 w261 w278 w295]
          tunnel: w201 -> [_ w209 w226 w243 w260 w277 w294]
          tunnel: "修改模式" -> [_ w207 w224 w241 w258 w275 w292]
          frame Default {
          }
          frame "cfg_False" {
            n77 = case shown="\"单独修改各状态\"" w207 {
              tunnel: [i32[] [0] ("Update Index") i32[] [0, 2, 4] ("Update Index") i32[] [0, 1, 2, 3, 4, 5] ("Update Index")] -> w208
              frame "单独修改各状态" {
              }
              frame "统一修改T/F状态" {
              }
              frame "统一修改全部状态" {
              }
            }
            n78 = for {
              tunnel: w209 -> [w217]
              shift-right: [w219] -> w211
              shift-left: w210 -> [w218]
              tunnel: [w216] -> w206
              tunnel: w208 -> [w215] mode=indexing
              n79 = call "_CSTK_Button_Icon_Config_UpdateConfiguration.vi"("Update Index"=w215, "Configuration in"=w217, "State 输入"=w218) -> ("Configuration out"=w216:T20, "State 输出"=w219:T1)  [unwired: 6 in, 1 out]
            }
            n80 = case shown="\"单独修改各状态\"" w207 {
              tunnel: w206 -> [w212 w213 w214]
              frame "单独修改各状态" {
                n81 = property on="cfg_False" class="Clust (严格)"("Value"=w212) -> ()  [unwired: 2 in, 2 out]
              }
              frame "统一修改T/F状态" {
                n82 = property on="cfg_False" class="Clust (严格)"("Value"=w213) -> ()  [unwired: 2 in, 2 out]
                n83 = property on="cfg_TrueToFalse" class="Clust (严格)"("Value"=w213) -> ()  [unwired: 2 in, 2 out]
                n84 = property on="cfg_HoverInFalse" class="Clust (严格)"("Value"=w213) -> ()  [unwired: 2 in, 2 out]
              }
              frame "统一修改全部状态" {
                n85 = property on="cfg_False" class="Clust (严格)"("Value"=w214) -> ()  [unwired: 2 in, 2 out]
                n86 = property on="cfg_True" class="Clust (严格)"("Value"=w214) -> ()  [unwired: 2 in, 2 out]
                n87 = property on="cfg_TrueToFalse" class="Clust (严格)"("Value"=w214) -> ()  [unwired: 2 in, 2 out]
                n88 = property on="cfg_FalseToTrue" class="Clust (严格)"("Value"=w214) -> ()  [unwired: 2 in, 2 out]
                n89 = property on="cfg_HoverInFalse" class="Clust (严格)"("Value"=w214) -> ()  [unwired: 2 in, 2 out]
                n90 = property on="cfg_HoverInTrue" class="Clust (严格)"("Value"=w214) -> ()  [unwired: 2 in, 2 out]
              }
            }
          }
          frame "cfg_True" {
            n91 = case shown="\"单独修改各状态\"" w224 {
              tunnel: [i32[] [1] ("Update Index") i32[] [1, 3, 5] ("Update Index") i32[] [0, 1, 2, 3, 4, 5] ("Update Index")] -> w225
              frame "单独修改各状态" {
              }
              frame "统一修改T/F状态" {
              }
              frame "统一修改全部状态" {
              }
            }
            n92 = for {
              tunnel: w226 -> [w234]
              shift-right: [w236] -> w228
              shift-left: w227 -> [w235]
              tunnel: [w233] -> w223
              tunnel: w225 -> [w232] mode=indexing
              n93 = call "_CSTK_Button_Icon_Config_UpdateConfiguration.vi"("Update Index"=w232, "Configuration in"=w234, "State 输入"=w235) -> ("Configuration out"=w233:T20, "State 输出"=w236:T1)  [unwired: 6 in, 1 out]
            }
            n94 = case shown="\"单独修改各状态\"" w224 {
              tunnel: w223 -> [w229 w230 w231]
              frame "单独修改各状态" {
                n95 = property on="cfg_True" class="Clust (严格)"("Value"=w229) -> ()  [unwired: 2 in, 2 out]
              }
              frame "统一修改T/F状态" {
                n96 = property on="cfg_True" class="Clust (严格)"("Value"=w230) -> ()  [unwired: 2 in, 2 out]
                n97 = property on="cfg_FalseToTrue" class="Clust (严格)"("Value"=w230) -> ()  [unwired: 2 in, 2 out]
                n98 = property on="cfg_HoverInTrue" class="Clust (严格)"("Value"=w230) -> ()  [unwired: 2 in, 2 out]
              }
              frame "统一修改全部状态" {
                n99 = property on="cfg_False" class="Clust (严格)"("Value"=w231) -> ()  [unwired: 2 in, 2 out]
                n100 = property on="cfg_True" class="Clust (严格)"("Value"=w231) -> ()  [unwired: 2 in, 2 out]
                n101 = property on="cfg_TrueToFalse" class="Clust (严格)"("Value"=w231) -> ()  [unwired: 2 in, 2 out]
                n102 = property on="cfg_FalseToTrue" class="Clust (严格)"("Value"=w231) -> ()  [unwired: 2 in, 2 out]
                n103 = property on="cfg_HoverInFalse" class="Clust (严格)"("Value"=w231) -> ()  [unwired: 2 in, 2 out]
                n104 = property on="cfg_HoverInTrue" class="Clust (严格)"("Value"=w231) -> ()  [unwired: 2 in, 2 out]
              }
            }
          }
          frame "cfg_TrueToFalse" {
            n105 = case shown="\"单独修改各状态\"" w241 {
              tunnel: [i32[] [2] ("Update Index") i32[] [0, 2, 4] ("Update Index") i32[] [0, 1, 2, 3, 4, 5] ("Update Index")] -> w242
              frame "单独修改各状态" {
              }
              frame "统一修改T/F状态" {
              }
              frame "统一修改全部状态" {
              }
            }
            n106 = for {
              tunnel: w243 -> [w251]
              shift-right: [w253] -> w245
              shift-left: w244 -> [w252]
              tunnel: [w250] -> w240
              tunnel: w242 -> [w249] mode=indexing
              n107 = call "_CSTK_Button_Icon_Config_UpdateConfiguration.vi"("Update Index"=w249, "Configuration in"=w251, "State 输入"=w252) -> ("Configuration out"=w250:T20, "State 输出"=w253:T1)  [unwired: 6 in, 1 out]
            }
            n108 = case shown="\"单独修改各状态\"" w241 {
              tunnel: w240 -> [w246 w247 w248]
              frame "单独修改各状态" {
                n109 = property on="cfg_TrueToFalse" class="Clust (严格)"("Value"=w246) -> ()  [unwired: 2 in, 2 out]
              }
              frame "统一修改T/F状态" {
                n110 = property on="cfg_False" class="Clust (严格)"("Value"=w247) -> ()  [unwired: 2 in, 2 out]
                n111 = property on="cfg_TrueToFalse" class="Clust (严格)"("Value"=w247) -> ()  [unwired: 2 in, 2 out]
                n112 = property on="cfg_HoverInFalse" class="Clust (严格)"("Value"=w247) -> ()  [unwired: 2 in, 2 out]
              }
              frame "统一修改全部状态" {
                n113 = property on="cfg_False" class="Clust (严格)"("Value"=w248) -> ()  [unwired: 2 in, 2 out]
                n114 = property on="cfg_True" class="Clust (严格)"("Value"=w248) -> ()  [unwired: 2 in, 2 out]
                n115 = property on="cfg_TrueToFalse" class="Clust (严格)"("Value"=w248) -> ()  [unwired: 2 in, 2 out]
                n116 = property on="cfg_FalseToTrue" class="Clust (严格)"("Value"=w248) -> ()  [unwired: 2 in, 2 out]
                n117 = property on="cfg_HoverInFalse" class="Clust (严格)"("Value"=w248) -> ()  [unwired: 2 in, 2 out]
                n118 = property on="cfg_HoverInTrue" class="Clust (严格)"("Value"=w248) -> ()  [unwired: 2 in, 2 out]
              }
            }
          }
          frame "cfg_FalseToTrue" {
            n119 = case shown="\"单独修改各状态\"" w258 {
              tunnel: [i32[] [3] ("Update Index") i32[] [1, 3, 5] ("Update Index") i32[] [0, 1, 2, 3, 4, 5] ("Update Index")] -> w259
              frame "单独修改各状态" {
              }
              frame "统一修改T/F状态" {
              }
              frame "统一修改全部状态" {
              }
            }
            n120 = for {
              tunnel: w260 -> [w268]
              shift-right: [w270] -> w262
              shift-left: w261 -> [w269]
              tunnel: [w267] -> w257
              tunnel: w259 -> [w266] mode=indexing
              n121 = call "_CSTK_Button_Icon_Config_UpdateConfiguration.vi"("Update Index"=w266, "Configuration in"=w268, "State 输入"=w269) -> ("Configuration out"=w267:T20, "State 输出"=w270:T1)  [unwired: 6 in, 1 out]
            }
            n122 = case shown="\"单独修改各状态\"" w258 {
              tunnel: w257 -> [w263 w264 w265]
              frame "单独修改各状态" {
                n123 = property on="cfg_FalseToTrue" class="Clust (严格)"("Value"=w263) -> ()  [unwired: 2 in, 2 out]
              }
              frame "统一修改T/F状态" {
                n124 = property on="cfg_True" class="Clust (严格)"("Value"=w264) -> ()  [unwired: 2 in, 2 out]
                n125 = property on="cfg_FalseToTrue" class="Clust (严格)"("Value"=w264) -> ()  [unwired: 2 in, 2 out]
                n126 = property on="cfg_HoverInTrue" class="Clust (严格)"("Value"=w264) -> ()  [unwired: 2 in, 2 out]
              }
              frame "统一修改全部状态" {
                n127 = property on="cfg_False" class="Clust (严格)"("Value"=w265) -> ()  [unwired: 2 in, 2 out]
                n128 = property on="cfg_True" class="Clust (严格)"("Value"=w265) -> ()  [unwired: 2 in, 2 out]
                n129 = property on="cfg_TrueToFalse" class="Clust (严格)"("Value"=w265) -> ()  [unwired: 2 in, 2 out]
                n130 = property on="cfg_FalseToTrue" class="Clust (严格)"("Value"=w265) -> ()  [unwired: 2 in, 2 out]
                n131 = property on="cfg_HoverInFalse" class="Clust (严格)"("Value"=w265) -> ()  [unwired: 2 in, 2 out]
                n132 = property on="cfg_HoverInTrue" class="Clust (严格)"("Value"=w265) -> ()  [unwired: 2 in, 2 out]
              }
            }
          }
          frame "cfg_HoverInFalse" {
            n133 = case shown="\"单独修改各状态\"" w275 {
              tunnel: [i32[] [4] ("Update Index") i32[] [0, 2, 4] ("Update Index") i32[] [0, 1, 2, 3, 4, 5] ("Update Index")] -> w276
              frame "单独修改各状态" {
              }
              frame "统一修改T/F状态" {
              }
              frame "统一修改全部状态" {
              }
            }
            n134 = for {
              tunnel: w277 -> [w285]
              shift-right: [w287] -> w279
              shift-left: w278 -> [w286]
              tunnel: [w284] -> w274
              tunnel: w276 -> [w283] mode=indexing
              n135 = call "_CSTK_Button_Icon_Config_UpdateConfiguration.vi"("Update Index"=w283, "Configuration in"=w285, "State 输入"=w286) -> ("Configuration out"=w284:T20, "State 输出"=w287:T1)  [unwired: 6 in, 1 out]
            }
            n136 = case shown="\"单独修改各状态\"" w275 {
              tunnel: w274 -> [w280 w281 w282]
              frame "单独修改各状态" {
                n137 = property on="cfg_HoverInFalse" class="Clust (严格)"("Value"=w280) -> ()  [unwired: 2 in, 2 out]
              }
              frame "统一修改T/F状态" {
                n138 = property on="cfg_False" class="Clust (严格)"("Value"=w281) -> ()  [unwired: 2 in, 2 out]
                n139 = property on="cfg_TrueToFalse" class="Clust (严格)"("Value"=w281) -> ()  [unwired: 2 in, 2 out]
                n140 = property on="cfg_HoverInFalse" class="Clust (严格)"("Value"=w281) -> ()  [unwired: 2 in, 2 out]
              }
              frame "统一修改全部状态" {
                n141 = property on="cfg_False" class="Clust (严格)"("Value"=w282) -> ()  [unwired: 2 in, 2 out]
                n142 = property on="cfg_True" class="Clust (严格)"("Value"=w282) -> ()  [unwired: 2 in, 2 out]
                n143 = property on="cfg_TrueToFalse" class="Clust (严格)"("Value"=w282) -> ()  [unwired: 2 in, 2 out]
                n144 = property on="cfg_FalseToTrue" class="Clust (严格)"("Value"=w282) -> ()  [unwired: 2 in, 2 out]
                n145 = property on="cfg_HoverInFalse" class="Clust (严格)"("Value"=w282) -> ()  [unwired: 2 in, 2 out]
                n146 = property on="cfg_HoverInTrue" class="Clust (严格)"("Value"=w282) -> ()  [unwired: 2 in, 2 out]
              }
            }
          }
          frame "cfg_HoverInTrue" {
            n147 = case shown="\"单独修改各状态\"" w292 {
              tunnel: [i32[] [5] ("Update Index") i32[] [1, 3, 5] ("Update Index") i32[] [0, 1, 2, 3, 4, 5] ("Update Index")] -> w293
              frame "单独修改各状态" {
              }
              frame "统一修改T/F状态" {
              }
              frame "统一修改全部状态" {
              }
            }
            n148 = for {
              tunnel: w294 -> [w302]
              shift-right: [w304] -> w296
              shift-left: w295 -> [w303]
              tunnel: [w301] -> w291
              tunnel: w293 -> [w300] mode=indexing
              n149 = call "_CSTK_Button_Icon_Config_UpdateConfiguration.vi"("Update Index"=w300, "Configuration in"=w302, "State 输入"=w303) -> ("Configuration out"=w301:T20, "State 输出"=w304:T1)  [unwired: 6 in, 1 out]
            }
            n150 = case shown="\"单独修改各状态\"" w292 {
              tunnel: w291 -> [w297 w298 w299]
              frame "单独修改各状态" {
                n151 = property on="cfg_HoverInTrue" class="Clust (严格)"("Value"=w297) -> ()  [unwired: 2 in, 2 out]
              }
              frame "统一修改T/F状态" {
                n152 = property on="cfg_True" class="Clust (严格)"("Value"=w298) -> ()  [unwired: 2 in, 2 out]
                n153 = property on="cfg_FalseToTrue" class="Clust (严格)"("Value"=w298) -> ()  [unwired: 2 in, 2 out]
                n154 = property on="cfg_HoverInTrue" class="Clust (严格)"("Value"=w298) -> ()  [unwired: 2 in, 2 out]
              }
              frame "统一修改全部状态" {
                n155 = property on="cfg_False" class="Clust (严格)"("Value"=w299) -> ()  [unwired: 2 in, 2 out]
                n156 = property on="cfg_True" class="Clust (严格)"("Value"=w299) -> ()  [unwired: 2 in, 2 out]
                n157 = property on="cfg_TrueToFalse" class="Clust (严格)"("Value"=w299) -> ()  [unwired: 2 in, 2 out]
                n158 = property on="cfg_FalseToTrue" class="Clust (严格)"("Value"=w299) -> ()  [unwired: 2 in, 2 out]
                n159 = property on="cfg_HoverInFalse" class="Clust (严格)"("Value"=w299) -> ()  [unwired: 2 in, 2 out]
                n160 = property on="cfg_HoverInTrue" class="Clust (严格)"("Value"=w299) -> ()  [unwired: 2 in, 2 out]
              }
            }
          }
        }
        n161 = Generate User Event(user event=w198, event data cluster=T23 {"Action"="UpdateImg", "Value"=variant, "Remark"=""} ("事件数据"), error in=w196) -> (error out=w195:errorcluster)  [unwired: 1 in, 1 out]
      }
    }
  }
  "State out" <- w1
  "State Changed?" <- w13
  "Action Name" <- w11
  n162 = Unregister For Events(event registration refnum=w16, error in=w15) -> (error out=w17:errorcluster)
  n163 = Destroy User Event(user event=w14, error in=w17) -> (error out=w6:errorcluster)
  n164 = invoke class="VI" method="FP.Close"(reference=w5, error in=w6) -> ()  [unwired: 1 in, 3 out]
